vi "Set USIM XOR Res Length.vi"(8 "error in (no error)":errorcluster, 9 "Length (Any)":i32(ring) items=["Any", "L04", "L05", "L06", "L07", "L08", "L09", "L10", "L11", "L12", "L13", "L14", "L15", "L16"], 10 "SIM Profile (\"SIM1\")":string="SIM1", 11 "VISA resource name":refnum<visa-resource-name>) -> (0 "error out":errorcluster, 3 "VISA resource name out":refnum<visa-resource-name>)   [LabVIEW 2020, in "Rohde&Schwarz CMXP Base.lvlib"]
doc: "Specifies the length of the RES (L2) for XOR authentication algorithms.\n\nAttribute:\n-\n\nRemote-control command:\n[CONFigure:]SIMProfile:USIM:SECurity:XORLength"
uses:
  <instrlib>/Rohde&Schwarz CMXP Base/Rohde&Schwarz CMXP Base.lvlib
  <instrlib>/Rohde&Schwarz CMXP Base/Private/rsidr_core.llb/rsidr_core.lvlib
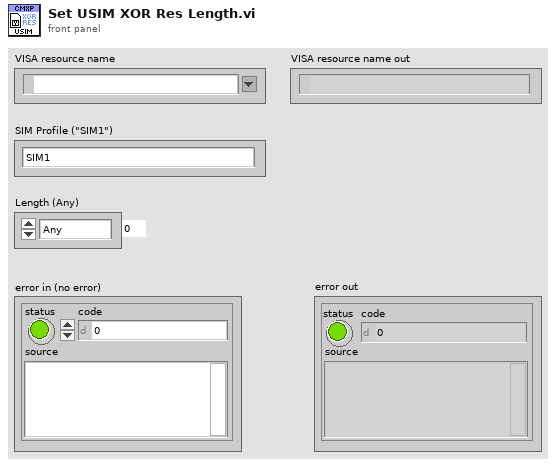
[diagram p1: front panel]
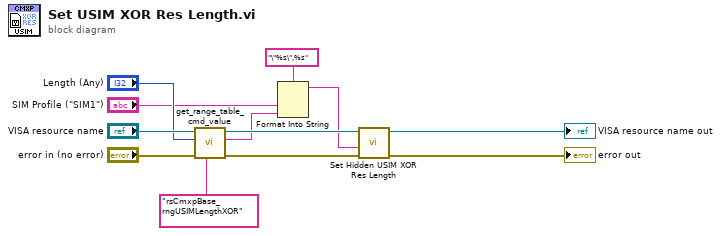
[diagram p0: block diagram]
diagram:
  n1 = call <instrlib>:"get_range_table_cmd_value.vi"("Range Table ID in"="rsCmxpBase_rngUSIMLengthXOR", "error in"="error in (no error)", "Input Int32 value"="Length (Any)", "VISA resource name"="VISA resource name") -> ("error out"=w3:errorcluster, "Cmd value out"=w1:string, "VISA resource name out"=w5:refnum<visa-resource-name>)  [unwired: 5 in]
  n2 = Format Into String(format string="\"%s\",%s", "SIM Profile (\"SIM1\")", w1) -> (resulting string=w2:string)  [unwired: 2 in, 1 out]
  n3 = call "Set Hidden USIM XOR Res Length"("error in (no error)"=w3, "Hidden USIM XOR Res Length ()"=w2, "instrument handle"=w5) -> ("error out"=→"error out":errorcluster, "instrument handle out"=→"VISA resource name out":refnum<visa-resource-name>)  [unwired: 7 in]
